vi "_QMH_Dequeue.vi"(8 "error in (no error)":errorcluster, 10 "timeout in ms (-1)":i32=-1, 11 "QMH in":refnum<class "QMH.lvclass">) -> (0 "error out":errorcluster, 1 "Data":variant, 2 "Msg":string, 3 "QMH out":refnum<class "QMH.lvclass">, 4 "timed out?":bool, 5 "# elements in queue":i32)   [LabVIEW 2018, in "QMH.lvclass"]
uses:
  QMH.lvclass
  QMH.lvclass/QMH.ctl
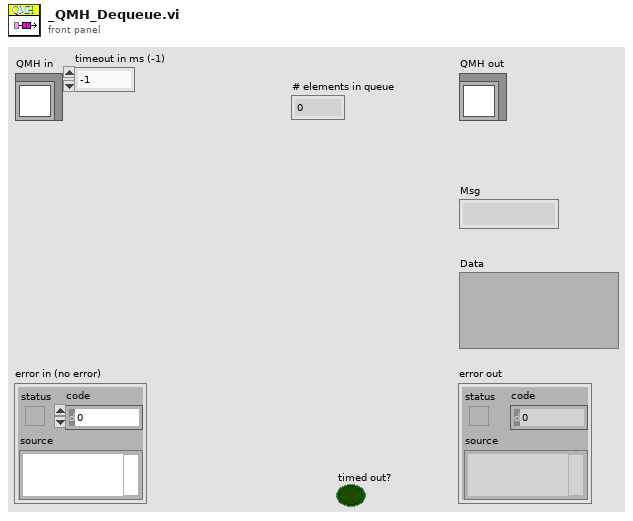
[diagram p1: front panel]
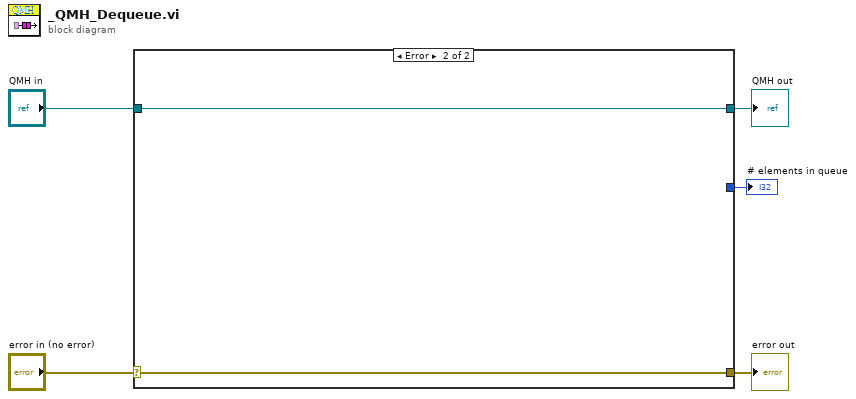
[diagram p0: block diagram]
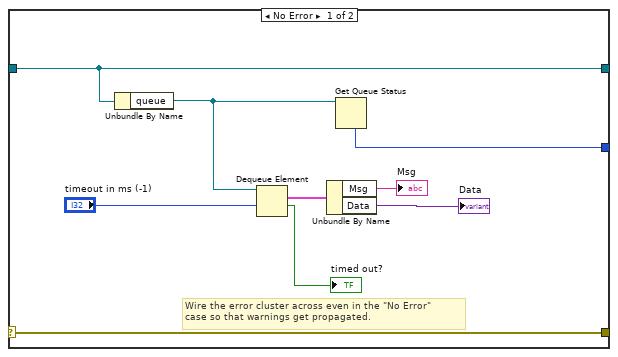
[diagram p2: hidden frame]
diagram:
  n1 = case shown="Error" "error in (no error)" {
    selector: "error in (no error)" -> [w14 w16]
    tunnel: [w14 w16] -> w4
    tunnel: [w13 w15] -> w2
    tunnel: "QMH in" -> [w13 w15]
    tunnel: [w6 _] -> w1
    frame No Error {
      # "Wire the error cluster across even in the \"No Error\"\ncase so that warnings get propagated."
      n2 = Unbundle By Name(w13) -> ("queue"=w7:refnum<queue>)
      n3 = Dequeue Element(queue=w7, timeout in ms (-1)="timeout in ms (-1)") -> (element=w11:cluster{"Data":variant, "Msg":string}, timed out?=→"timed out?":bool)  [unwired: 1 in, 2 out]
      n4 = Unbundle By Name(w11) -> ("Msg"=→"Msg":string, "Data"=→"Data":variant)
      n5 = Get Queue Status(queue=w7) -> (# elements in queue=w6:i32)  [unwired: 2 in, 7 out]
    }
    frame Error {
    }
  }
  "error out" <- w4
  "QMH out" <- w2
  "# elements in queue" <- w1
